vi "radial-profile-xyR-range-from2DarrayDBL.vi"(4 "R-max":sgl, 5 "num":i32=2, 6 "R-min":sgl, 7 "R-step":sgl=1.0, 8 "error in (no error)":errorcluster caption="错误输入（无错误）", 10 "y/x":dbl[](array[numeric]), 11 "2D array":dbl[][](array[numeric])) -> (0 "error out":errorcluster caption="错误输出", 1 "ArrayR":sgl[](array[numeric]), 2 "profile":dbl[](array[numeric]))   [LabVIEW 2013]
panel:
  in  "method":i32(ring)=3 items=["nearest", "bilinear", "bicubic", "bicubic spline"]
  # "Because the center-symetric property of power spectrum (fft) of images, \nwe use pi instead of 2pi, \nand set num=2 to cut the calculation time by 50%."
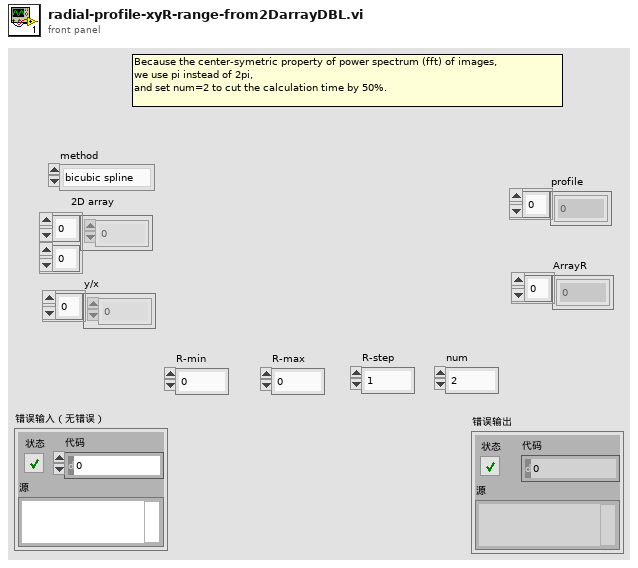
[diagram p1: front panel]
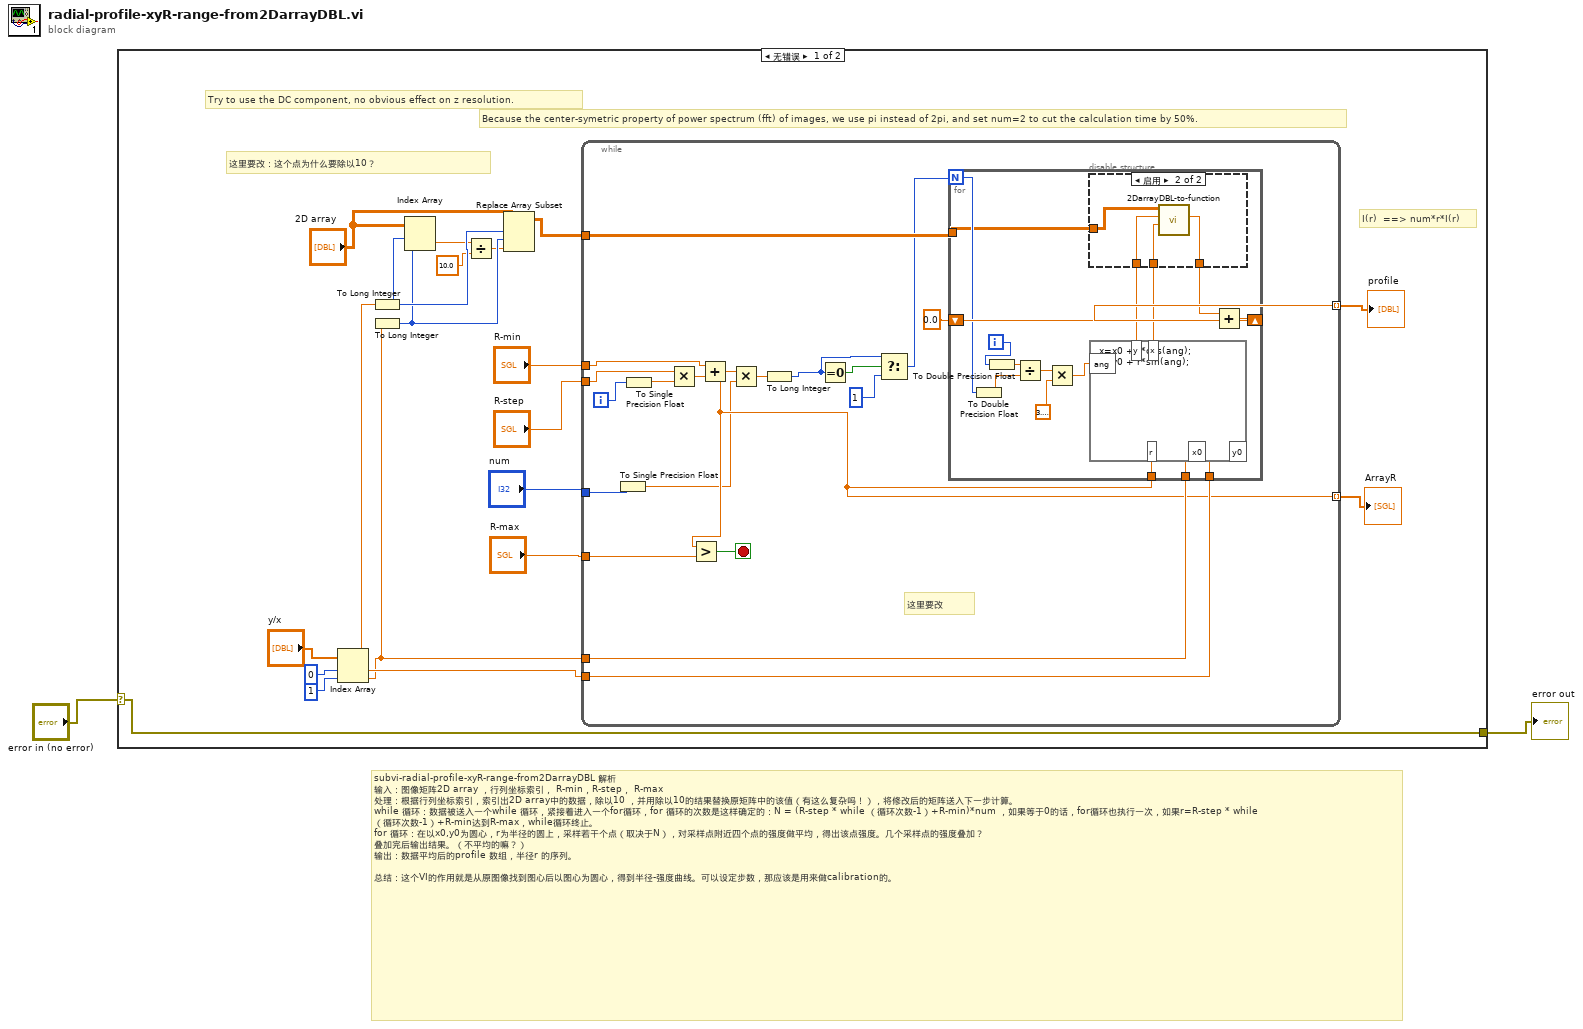
[diagram p0: block diagram]
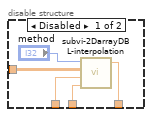
[diagram p2: hidden frame]
diagram:
  # "subvi-radial-profile-xyR-range-from2DarrayDBL 解析\n输入：图像矩阵2D array ，行列坐标索引， R-min，R-step， R-max\n处理：根据行列坐标索引，索引出2D array中的数据，除以10 ，并用除以10的结果替换原矩阵中的该值（有这么复杂吗！），将修改后的矩阵送入下一步计算。\nwhile 循环：数据被送入一个while 循环，紧接着进入一个for循环，for 循环的次数是这样确定的：N = (R-step * while （循环次数-1）+R-min)*num ，如果等于0的话，for循环也执行一次，如果r=R-step * while （循环次数-1）+R-min达到R-max，while循环终止。\nfor 循环：在以x0,y0为圆心，r为半径的圆上，采样若干个点（取决于N），对采样点附近四个点的强度做平均，得出该点强度。几个采样点的强度叠加？\n叠加完后输出结果。（不平均的嘛？）\n输出：数据平均后的profile 数组，半径r 的序列。\n\n总结：这个VI的作用就是从原图像找到图心后以图心为圆心，得到半径-强度曲线。可以设定步数，那应该是用来做calibration的。"
  n1 = case shown="无错误" "error in (no error)" {
    selector: "error in (no error)" -> [w3 w67]
    tunnel: [w3 w67] -> w1
    frame No Error {
      # "这里要改：这个点为什么要除以10？"
      # "Try to use the DC component, no obvious effect on z resolution."
      # "I(r)  ==> num*r*I(r)"
      # "Because the center-symetric property of power spectrum (fft) of images, we use pi instead of 2pi, and set num=2 to cut the calculation time by 50%."
      n2 = Index Array(array="y/x", index #1=0 ("index"), index #2=1 ("index")) -> (element #1=w12:dbl, element #2=w11:dbl)
      n3 = To Long Integer(number=w12) -> (32bit integer=w9:i32)
      n4 = To Long Integer(number=w11) -> (32bit integer=w8:i32)
      n5 = Index Array(array="2D array", index (row)=w9, index (col)=w8) -> (element=w7:dbl)
      n6 = Divide(x=w7, y=10.0) -> (x/y=w5:dbl)
      n7 = Replace Array Subset(array="2D array", new element=w5, index (row)=w9, index (col)=w8) -> (w4:dbl[][])
      n8 = while {
        tunnel: w4 -> [w41]
        tunnel: [w28] -> w14 mode=indexing
        tunnel: w12 -> [w39]
        tunnel: w11 -> [w38]
        tunnel: "R-step" -> [w34]
        tunnel: "R-min" -> [w37]
        tunnel: "R-max" -> [w32]
        tunnel: "num" -> [w31]
        tunnel: [w29] -> w13 mode=indexing
        i -> [w35]
        stop <- w33 stop-if-true
        # "这里要改"
        n9 = To Single Precision Float(number=w31) -> (single precision float=w22:sgl)
        n10 = To Single Precision Float(number=w35) -> (single precision float=w23:sgl)
        n11 = Multiply(x=w34, y=w23) -> (x*y=w36:sgl)
        n12 = Add(x=w37, y=w36) -> (x+y=w29:sgl)
        n13 = Greater?(x=w29, y=w32) -> (0:w33:bool)
        n14 = Multiply(x=w29, y=w22) -> (x*y=w30:sgl)
        n15 = To Long Integer(number=w30) -> (32bit integer=w26:i32)
        n16 = Equal To 0?(x=w26) -> (x = 0?=w27:bool)
        n17 = Select(t=w26, s=w27, f=1) -> (s? t:f=w24:i32)
        n18 = for {
          N: w24 -> [w50]
          tunnel: w41 -> [w47]
          tunnel: w38 -> [w57]
          tunnel: w39 -> [w56]
          shift-right: [w51] -> w28
          shift-left: 0.0 -> [w52]
          tunnel: w29 -> [w49]
          i -> [w55]
          n19 = To Double Precision Float(number=w50) -> (double precision float=w42:dbl)
          n20 = To Double Precision Float(number=w55) -> (double precision float=w43:dbl)
          n21 = Divide(x=w43, y=w42) -> (x/y=w54:dbl)
          n22 = Multiply(x=w54, y=3.141592653589793) -> (x*y=w53:dbl)
          n23 = formula code="x=x0 + r*cos(ang);\ny=y0 + r*sin(ang);"("x0"=w57, "y0"=w56, "ang"=w53, "r"=w49) -> ("x"=w45:dbl, "y"=w46:dbl)
          n24 = disable-structure shown="启用" {
            disable-tunnel: w47 -> [w62 w66]
            disable-tunnel: w46 -> [w61 w65]
            disable-tunnel: w45 -> [w60 w64]
            disable-tunnel: [w59 w63] -> w44
            frame Disabled {
              n25 = call "subvi-2DarrayDBL-interpolation.vi"("xi"=w60, "yi"=w61, "2D array"=w62, "method"="method") -> ("f(x,y)"=w59:dbl)  [unwired: 2 out]
            }
            frame Enabled {
              n26 = call "2DarrayDBL-to-function.vi"("X"=w64, "Y"=w65, "2D array"=w66) -> ("f(x,y)"=w63:dbl)  [unwired: 6 in, 2 out]
            }
          }
          n27 = Add(x=w44, y=w52) -> (x+y=w51:dbl)
        }
      }
      "profile" <- w14
      "ArrayR" <- w13
    }
    frame Error {
    }
  }
  "error out" <- w1
